vi "Scale.vi"(8 "error in":errorcluster, 11 "INI file path":path=path "C:/Users/user/Documents/GitHub/AADXB08/AADXB08_LV/data/AADXB08.ini") -> (1 "min":dbl, 3 "Max":dbl)   [LabVIEW 2019]
uses:
  <vilib>/Utility/config.llb/Read Key (Double).vi
  <vilib>/Utility/config.llb/NI_LVConfig.lvlib
panel:
  out "error out":errorcluster
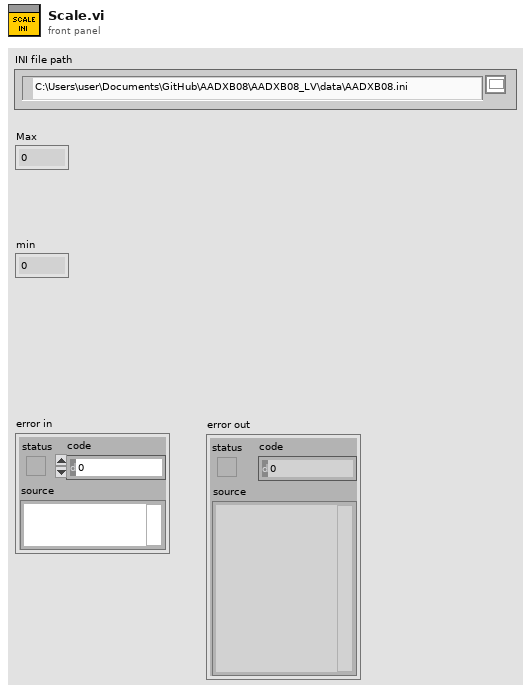
[diagram p1: front panel]
types:
  T1 = typedef "NI_LVConfig.lvlib/Config Data RefNum.ctl" = refnum<k1>
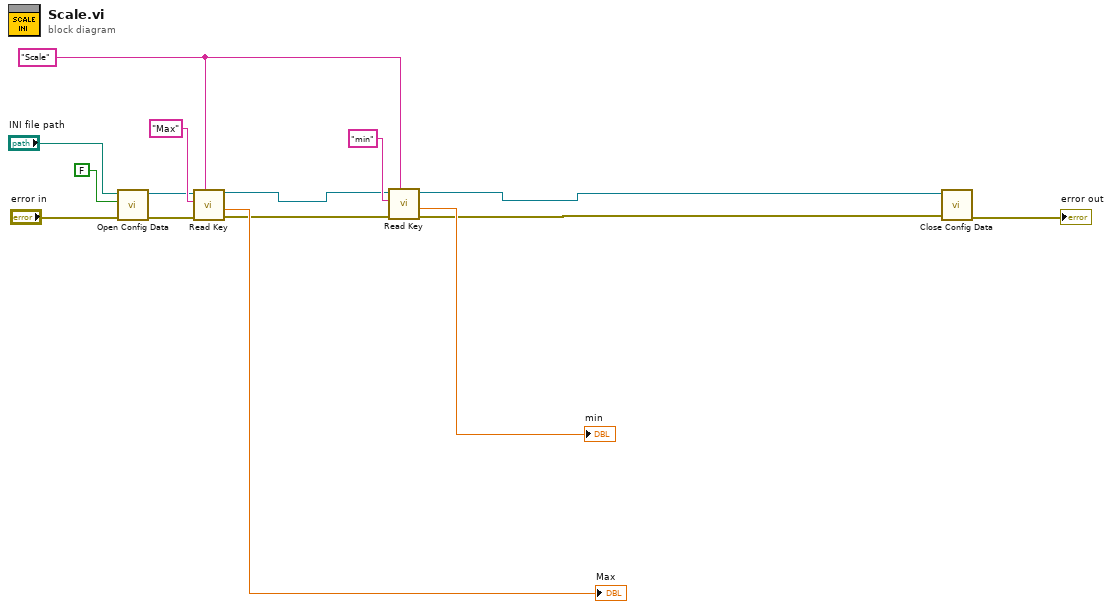
[diagram p0: block diagram]
diagram:
  w5 = "Scale" ("Main section")
  n1 = call <vilib>:"Open Config Data.vi"("error in (no error)"="error in", "create file if necessary (T)"=FALSE ("create file if necessary? (T)"), "configuration file path"="INI file path") -> ("error out"=w13:errorcluster, "refnum"=w11:T1)  [unwired: 6 in, 1 out]
  n2 = call-poly <vilib>:"Read Key.vi"("section"=w5, "error in (no error)"=w13, "key"="Max", "refnum"=w11) -> ("error out"=w3:errorcluster, "value"=→"Max":dbl, "refnum out"=w4:T1)  [unwired: 1 in, 4 out]
  n3 = call-poly <vilib>:"Read Key.vi"("section"=w5, "error in (no error)"=w3, "key"="min", "refnum"=w4) -> ("error out"=w1:errorcluster, "value"=→"min":dbl, "refnum out"=w2:T1)  [unwired: 1 in, 4 out]
  n4 = call <vilib>:"Close Config Data.vi"("error in (no error)"=w1, "refnum"=w2) -> ("error out"=→"error out":errorcluster)  [unwired: 1 in, 8 out]
